vi "Main.vi"(11 "Module Admin":refnum<class "Delacor_lib_QMH_Module Admin.lvclass">) -> ()   [LabVIEW 2023, in "Registration.lvlib"]
doc: "This template is based off of the Queued Message Handler design pattern and the Queued Message Handler project template that ships with LabVIEW.\n\nThe main difference is that the queue is private to this module and communication between modules is performed via Broadcast and Request events.\n\nRequest events are wrapped in public API methods and are handled in the Event Handling Loop (EHL) of this VI. Any module can register for Broadcast events sent by this module. The EHL generates messages based on user interface actions.\n\nThe Message Handling Loop (MHL) processes messages generated by the EHL, or by other messages. The messages are string values, so new messages can be added easily to the Message Cases case structure in the MHL. Each message cluster can also provide an optional value for Message Data, which is a variant that can be converted to whatever message-specific data is required.\n_____\nBased on DQMH Project Template 6.1.0.94."
uses:
  Registration.lvlib
  <vilib>/Delacor/Delacor QMH/Libraries/Module Admin_class/Delacor_lib_QMH_Module Admin.lvclass
  Data_reg.ctl
  Module Data--cluster.ctl
  Initial Data/InitalData Type.ctl
  <vilib>/Delacor/Delacor QMH/Libraries/Message Queue_class/Delacor_lib_QMH_Message Queue.lvclass/Delacor_lib_QMH_Message Queue.ctl
  Stop Argument--cluster.ctl
  <vilib>/Delacor/Delacor QMH/Libraries/Module Admin_class/Delacor_lib_QMH_Module Admin.lvclass/Delacor_lib_QMH_Module Admin.ctl
  New_Data Argument--cluster.ctl
  Send Main VI ref Argument--cluster.ctl
  <vilib>/Utility/miscctls.llb/LVPointTypeDef.ctl
  <vilib>/Delacor/Delacor QMH/Libraries/Message Queue_class/Delacor_lib_QMH_Enqueue Message (Single).vi
  <vilib>/Delacor/Delacor QMH/Libraries/Module Admin_class/Delacor_lib_QMH_Get External Launch.vi
  <vilib>/Utility/error.llb/Error Cluster From Error Code.vi
  <vilib>/Utility/file.llb/Write Delimited Spreadsheet (string).vi
  <vilib>/ErrorRing/Error Ring.xnode
  <vilib>/Delacor/Delacor QMH/Libraries/Message Queue_class/Delacor_lib_QMH_Message Queue.lvclass
  Initial Data/Initial Data.lvlib
panel:
  in  "open_F":bool
  in  "Registr start":bool
  in  "timeout":dbl=1.0 caption="Период регистрации" format="Период регистрации %#.1f сек"
  in  "set_path":bool
  out "file_path":string caption="Файл регистрации"
  out "error out":errorcluster
  in  "Simulate MHL Error":bool
  in  "Simulate EHL Error":bool
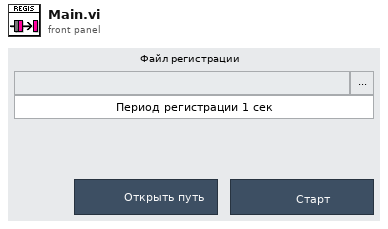
[diagram p1: front panel]
types:
  T1 = typedef "Registration.lvlib/Data_reg.ctl" = cluster{"Дата":string, "Время":string, "Рпл1, МПа":dbl, "Vпл, см3":dbl, "Рпл2, МПа":dbl, "Ргор, МПа":dbl, "Рэфф, МПа":dbl, "R, Ом":dbl, "dL, мм":dbl, "Ткд, градС":dbl, "Тпрод, мкс":dbl, "Тпоп.1, мкс":dbl, "Тпоп.2, мкс":dbl, "Рдм, МПа":dbl, "Q, мл":dbl, "Тнагр, градС":dbl, "ЦАП, градС":dbl}
  T2 = typedef "Registration.lvlib/Request Events--cluster.ctl" = cluster{"Stop Module":refnum<user-event>, "Show Panel":refnum<user-event>, "Hide Panel":refnum<user-event>, "Get Module Execution Status":refnum<user-event>, "Show Diagram":refnum<user-event>, "New_Data":refnum<user-event>, "Send Main VI ref":refnum<user-event>}
  T3 = typedef "Initial Data.lvlib/Broadcast Events--cluster.ctl" = cluster{"Module Did Init":refnum<user-event>, "Status Updated":refnum<user-event>, "Error Reported":refnum<user-event>, "Module Did Stop":refnum<user-event>, "Update Module Execution Status":refnum<user-event>, "Data":refnum<user-event>}
  T4 = typedef "Registration.lvlib/Module Data--cluster.ctl" = cluster{"reg_on":bool, "file_path":path, "Data reg":T1, "Исходные данные":T5}
  T5 = typedef "Initial Data.lvlib/InitalData Type.ctl" = cluster{"Дата":string, "Время":string, "Месторождение":string, "Пласт":string, "Скважина":string}
  T6 = enum32{"invalid lock state", "Not Locked", "Locked (No Password)", "Password-protected"}
  T7 = typedef "Registration.lvlib/Stop Argument--cluster.ctl" = cluster{"Origin":string, "Exit via Stop Module Req?":bool, "Wait for Module to stop?":bool}
  T8 = typedef "Registration.lvlib/New_Data Argument--cluster.ctl" = cluster{"Data reg":T1}
  T9 = typedef "Registration.lvlib/Send Main VI ref Argument--cluster.ctl" = cluster{"Boolean":bool}
  T10 = enum8{"Enabled", "Disabled", "Disabled and Grayed Out"}
  T11 = typedef "LVPointTypeDef.ctl" = cluster{"Horizontal":i16, "Vertical":i16}
  T12 = enum32{"Invalid", "Standard", "Closed", "Hidden", "Minimized", "Maximized"}
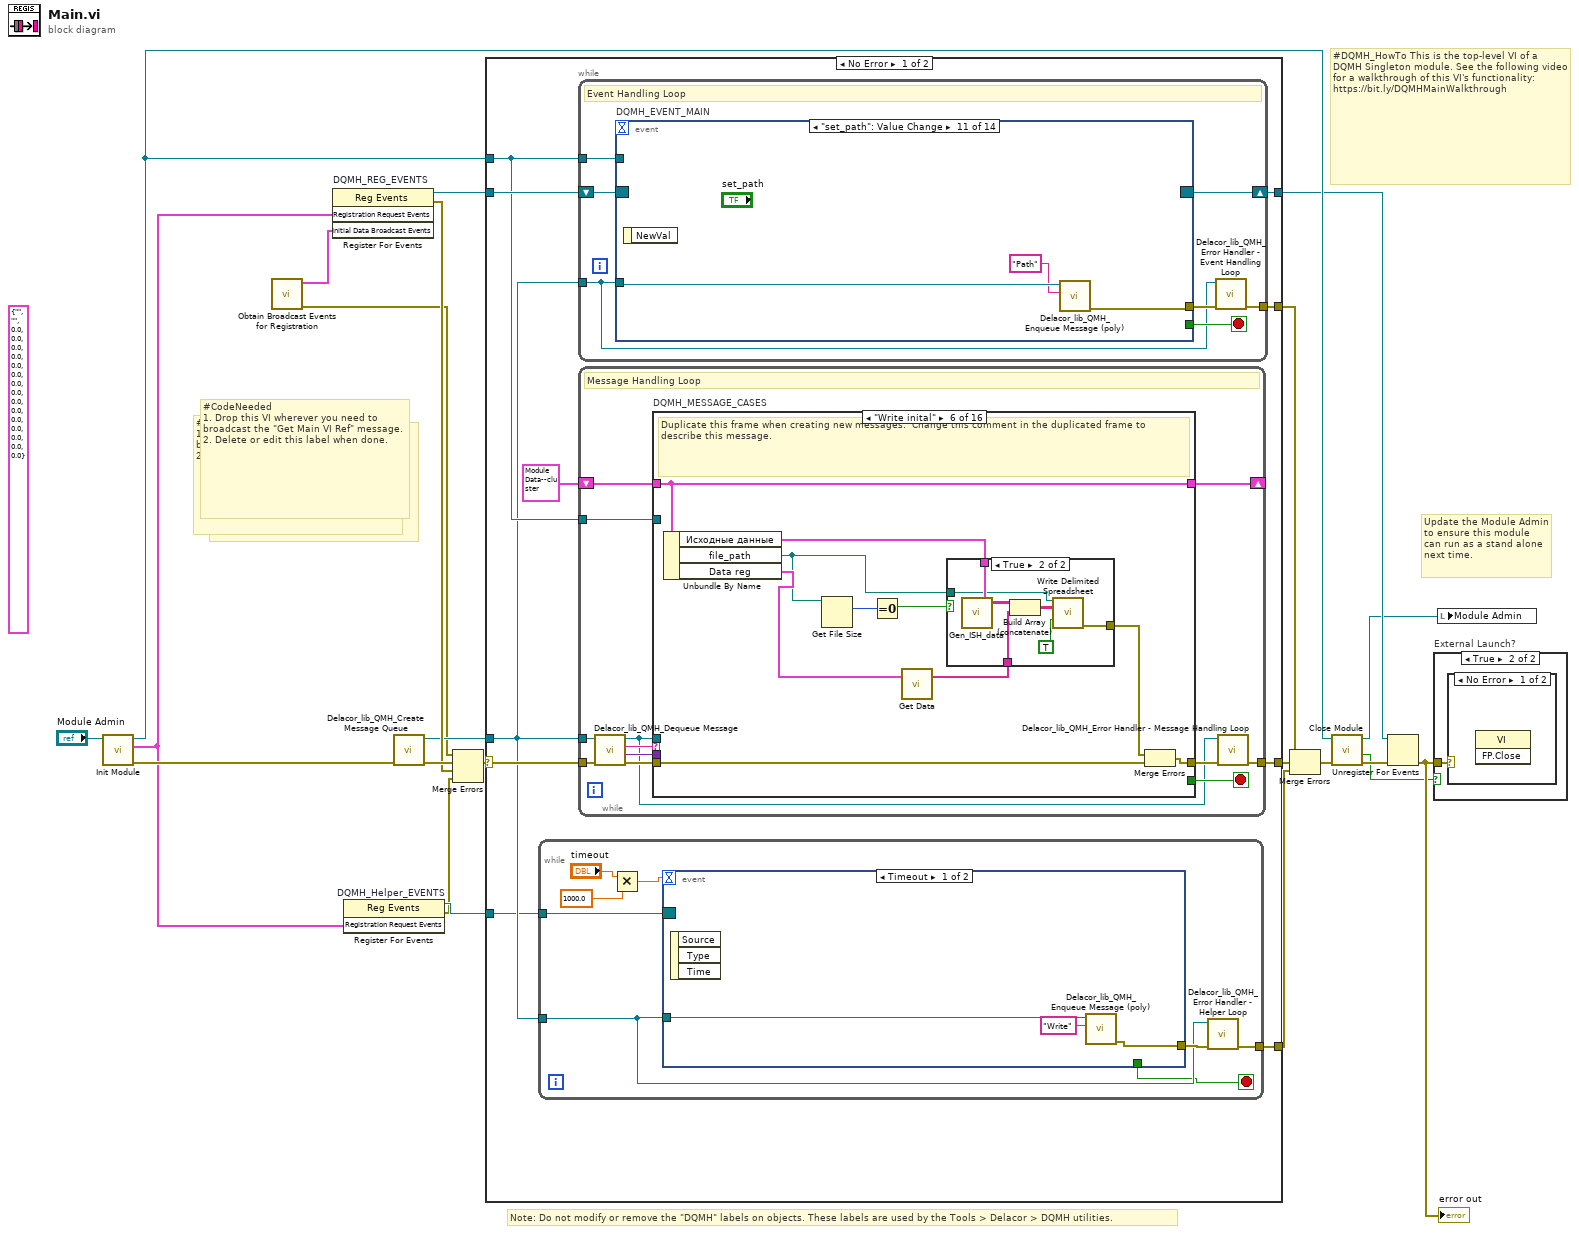
[diagram p0: block diagram]
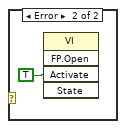
[diagram p3: hidden frame]
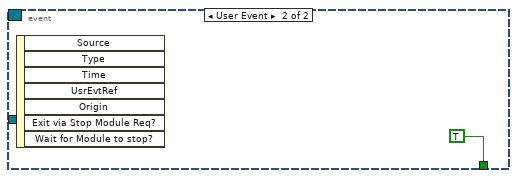
[diagram p4: hidden frame]
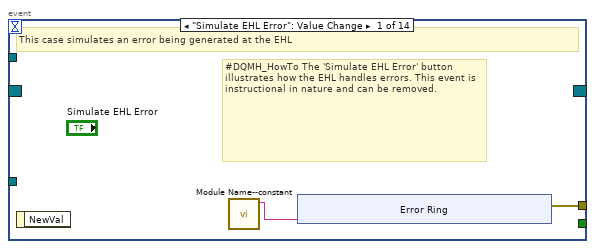
[diagram p5: hidden frame]
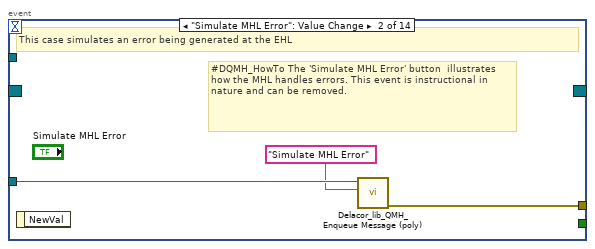
[diagram p6: hidden frame]
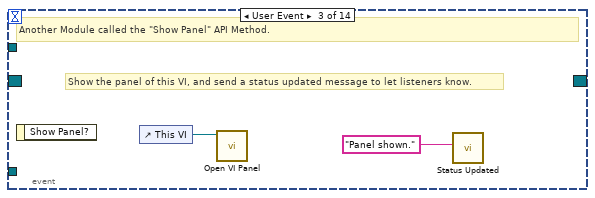
[diagram p7: hidden frame]
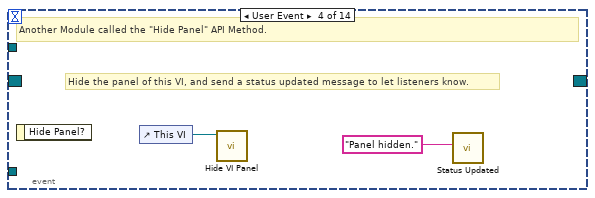
[diagram p8: hidden frame]
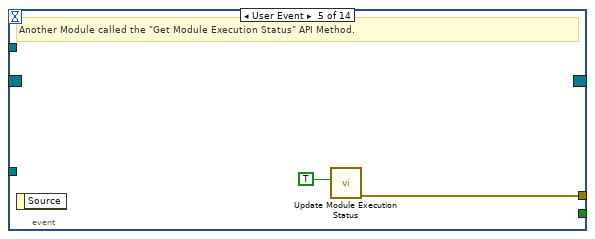
[diagram p9: hidden frame]
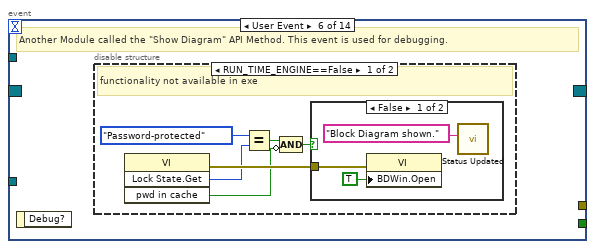
[diagram p10: hidden frame]
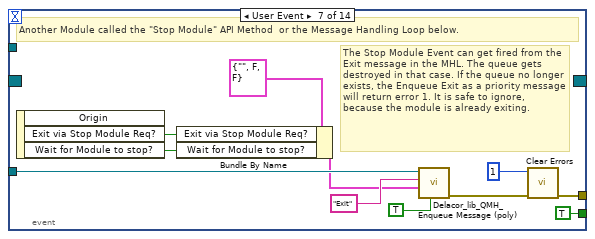
[diagram p13: hidden frame]
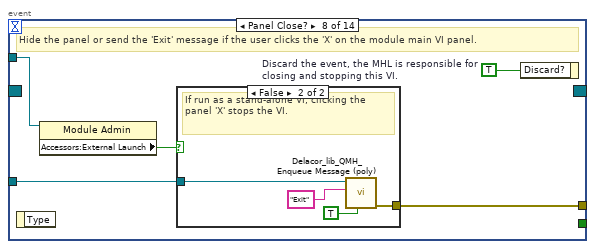
[diagram p14: hidden frame]
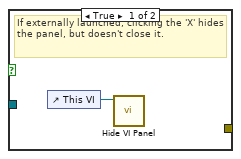
[diagram p15: hidden frame]
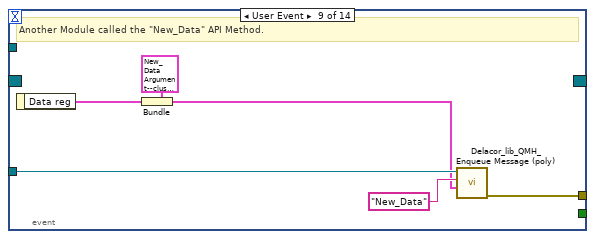
[diagram p16: hidden frame]
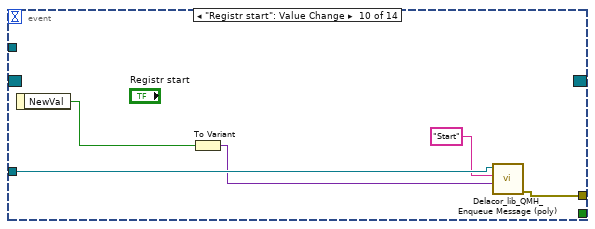
[diagram p17: hidden frame]
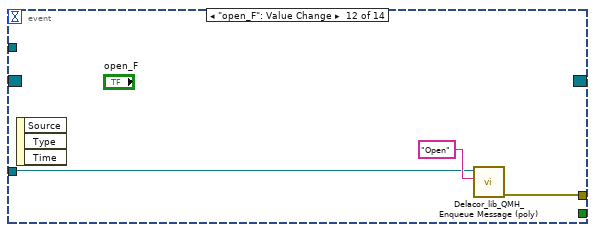
[diagram p18: hidden frame]
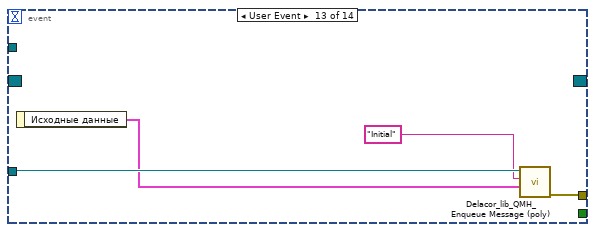
[diagram p19: hidden frame]
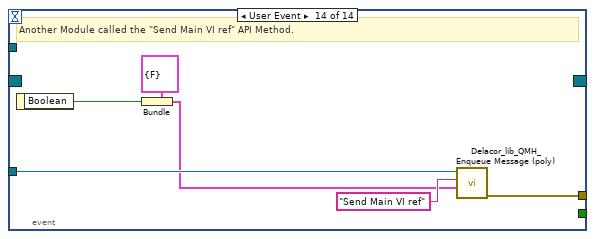
[diagram p20: hidden frame]
diagram:
  (unwired) T1 {"Дата"="", "Время"="", "Рпл1, МПа"=0.0, "Vпл, см3"=0.0, "Рпл2, МПа"=0.0, "Ргор, МПа"=0.0, "Рэфф, МПа"=0.0, "R, Ом"=0.0, "dL, мм"=0.0, "Ткд, градС"=0.0, "Тпрод, мкс"=0.0, "Тпоп.1, мкс"=0.0, "Тпоп.2, мкс"=0.0, "Рдм, МПа"=0.0, "Q, мл"=0.0, "Тнагр, градС"=0.0, "ЦАП, градС"=0.0} ("Data reg")
  # "#CodeNeeded\n1. Drop this VI wherever you need to broadcast the \"Get Main VI Reference\" message.\n2. Delete or edit this label when done."
  # "#CodeNeeded\n1. Drop this VI wherever you need to broadcast the \"Get Main VI Ref\" message.\n2. Delete or edit this label when done."
  # "#CodeNeeded\n1. Drop this VI wherever you need to broadcast the \"Get Main VI Ref\" message.\n2. Delete or edit this label when done."
  # "#DQMH_HowTo This is the top-level VI of a DQMH Singleton module. See the following video for a walkthrough of this VI's functionality: https://bit.ly/DQMHMainWalkthrough"
  # "Note: Do not modify or remove the \"DQMH\" labels on objects. These labels are used by the Tools > Delacor > DQMH utilities."
  # "Update the Module Admin to ensure this module can run as a stand alone next time."
  n1 = call "Init Module.vi"("Singleton Module Admin in"="Module Admin") -> ("error out"=w21:errorcluster, "Registration Request Events"=w1:T2, "Singleton Module Admin out"=w13:refnum<class "Delacor_lib_QMH_Module Admin.lvclass">)  [unwired: 8 in]
  n2 = call "Obtain Broadcast Events for Registration.vi"() -> ("error out"=w2:errorcluster, "Initial Data Broadcast Events"=w3:T3)  [unwired: 9 in, 1 out]
  n3 = register-events "DQMH_REG_EVENTS"(w1, w3) -> (reference out=w11:refnum<event-registration>, error out=w14:errorcluster)  [unwired: 2 in]
  n4 = register-events "DQMH_Helper_EVENTS"(w1) -> (reference out=w6:refnum<event-registration>, error out=w5:errorcluster)  [unwired: 2 in]
  n5 = call <vilib>:"Delacor_lib_QMH_Create Message Queue.vi"("error in"=w21) -> ("error out"=w16:errorcluster, "Message Queue"=w10:refnum<class "Delacor_lib_QMH_Message Queue.lvclass">)  [unwired: 9 in]
  n6 = Merge Errors(w2, w16, w14, w5) -> (w15:errorcluster)
  n7 = case shown="No Error" w15 {
    selector: w15 -> [w30 w340]
    tunnel: [w32 w339] -> w22
    tunnel: [w29 w345] -> w12
    tunnel: w11 -> [w27 w345]
    tunnel: w10 -> [w25 w338]
    tunnel: [w31 _] -> w19
    tunnel: w13 -> [w26 w341]
    tunnel: w6 -> [w24 _]
    tunnel: [w23 _] -> w4
    frame No Error {
      n8 = while {
        tunnel: w25 -> [w36]
        tunnel: w24 -> [w35]
        tunnel: [w33] -> w23
        stop <- w34 stop-if-true
        n9 = Multiply(x="timeout", y=1000.0) -> (x*y=w38:dbl)
        n10 = event shown="[0] Timeout" {
          selector: w35 -> [_ _]
          dyn-events: _ -> [_ _]
          timeout: w38 -> [_ _]
          tunnel: w36 -> [w43 _]
          tunnel: [w42 _] -> w37
          tunnel: [_ TRUE] -> w34
          event Timeout {
            n11 = event-data() -> ()  [unwired: 1 in, 3 out]
            n12 = call-poly <vilib>:"Delacor_lib_QMH_Enqueue Message (poly).vi"("Message"="Write", "Message Queue in"=w43) -> ("error out"=w42:errorcluster)  [unwired: 8 in, 1 out]
          }
          event User Event {
            n13 = event-data() -> ()  [unwired: 1 in, 7 out]
          }
        }
        n14 = call-dynamic "Delacor_lib_QMH_Error Handler - Helper Loop.vi"("error in"=w37, "Message Queue in"=w36) -> ("dup error in"=w33:errorcluster)  [unwired: 8 in, 1 out]
      }
      n15 = while {
        tunnel: w25 -> [w45]
        shift-right: [w48] -> w29
        shift-left: w27 -> [w49]
        tunnel: [w50] -> w31
        tunnel: w26 -> [w46]
        stop <- w47 stop-if-true
        # "Event Handling Loop"
        n16 = event "DQMH_EVENT_MAIN" shown="[10] \"set_path\": Value Change" {
          selector: w49 -> [_ _ _ _ _ _ _ _ _ _ _ _ _ _]
          dyn-events: [_ _ _ _ _ _ _ _ _ _ _ _ _ _] -> w48
          timeout: _ -> [_ _ _ _ _ _ _ _ _ _ _ _ _ _]
          tunnel: [_ _ _ _ _ _ TRUE ("Discard?") _ _ _ _ _ _ _] -> w47
          tunnel: w45 -> [_ w62 _ _ _ _ w85 w92 w105 w110 w112 w114 w119 w126]
          tunnel: [w53 w63 _ _ w69 _ w88 w94 w100 w109 w113 w115 w120 w121] -> w51
          tunnel: w46 -> [_ _ _ _ _ _ _ w91 _ _ _ _ _ _]
          event "Simulate EHL Error": Value Change {
            # "#DQMH_HowTo The 'Simulate EHL Error' button  illustrates how the EHL handles errors. This event is instructional in nature and can be removed."
            # "This case simulates an error being generated at the EHL"
            n17 = event-data() -> ()  [unwired: 1 in, 1 out]
            n18 = call "Module Name--constant.vi"() -> ("Module Name"=w52:string)  [unwired: 11 in]
            n19 = xnode "Error Ring"("parameter 0"=w52) -> ("error out"=w53:errorcluster)
          }
          event "Simulate MHL Error": Value Change {
            # "#DQMH_HowTo The 'Simulate MHL Error' button  illustrates how the MHL handles errors. This event is instructional in nature and can be removed."
            # "This case simulates an error being generated at the EHL"
            n20 = event-data() -> ()  [unwired: 1 in, 1 out]
            n21 = call-poly <vilib>:"Delacor_lib_QMH_Enqueue Message (poly).vi"("Message"="Simulate MHL Error", "Message Queue in"=w62) -> ("error out"=w63:errorcluster)  [unwired: 8 in, 1 out]
          }
          event User Event {
            # "Show the panel of this VI, and send a status updated message to let listeners know."
            # "Another Module called the \"Show Panel\" API Method."
            n22 = event-data() -> ()  [unwired: 1 in, 1 out]
            n23 = control-ref of="This VI"() -> (w65:refnum<vi>)
            n24 = call "Open VI Panel.vi"("VI"=w65) -> ()  [unwired: 10 in, 1 out]
            n25 = call "Status Updated.vi"("Status"="Panel shown." ("format string")) -> ()  [unwired: 10 in, 1 out]
          }
          event User Event {
            # "Hide the panel of this VI, and send a status updated message to let listeners know."
            # "Another Module called the \"Hide Panel\" API Method."
            n26 = event-data() -> ()  [unwired: 1 in, 1 out]
            n27 = control-ref of="This VI"() -> (w67:refnum<vi>)
            n28 = call "Hide VI Panel.vi"("VI"=w67) -> ()  [unwired: 10 in, 1 out]
            n29 = call "Status Updated.vi"("Status"="Panel hidden." ("format string")) -> ()  [unwired: 10 in, 1 out]
          }
          event User Event {
            # "Another Module called the \"Get Module Execution Status\" API Method."
            n30 = event-data() -> ()  [unwired: 1 in, 1 out]
            n31 = call "Update Module Execution Status.vi"("Running?"=TRUE) -> ("error out"=w69:errorcluster)  [unwired: 10 in]
          }
          event User Event {
            # "Another Module called the \"Show Diagram\" API Method. This event is used for debugging."
            n32 = event-data() -> ()  [unwired: 1 in, 1 out]
            n33 = disable-structure shown="RUN_TIME_ENGINE==False" {
              frame condition #0 (active) {
                # "functionality not available in exe"
                n34 = invoke class="VI" method="Lock State.Get"() -> (error out=w75:errorcluster, "Get Lock State"=w74:T6, "pwd in cache"=w71:bool)  [unwired: 4 in, 1 out]
                n35 = Equal?(x=T6."Password-protected", y=w74) -> (x = y?=w72:bool)
                n36 = Compound Arithmetic op=AND(w72, invert w71) -> (w70:bool)
                n37 = case shown="False" w70 {
                  tunnel: w75 -> [w78 _]
                  frame False {
                    n38 = property class="VI"(error in=w78, "BDWin.Open"=TRUE ("Block Diagram Window:Open")) -> ()  [unwired: 1 in, 2 out]
                    n39 = call "Status Updated.vi"("Status"="Block Diagram shown." ("format string")) -> ()  [unwired: 10 in, 1 out]
                  }
                  frame True {
                    # "Password-protected VI, and the password is not in the cache. Do not show the diagram."
                  }
                }
              }
              frame condition #1 {
              }
            }
          }
          event User Event {
            # "The Stop Module Event can get fired from the Exit message in the MHL. The queue gets destroyed in that case. If the queue no longer exists, the Enqueue Exit as a priority message will return error 1. It is safe to ignore, because the module is already exiting."
            # "Another Module called the \"Stop Module\" API Method  or the Message Handling Loop below."
            n40 = event-data() -> ("Exit via Stop Module Req?"=w81:bool, "Wait for Module to stop?"=w80:bool)  [unwired: 1 in, 1 out]
            n41 = Bundle By Name(cluster=T7 {"Origin"="", "Exit via Stop Module Req?"=FALSE, "Wait for Module to stop?"=FALSE} ("Stop Argument"), "Exit via Stop Module Req?"=w81, "Wait for Module to stop?"=w80) -> (w79:T7)
            n42 = call-poly <vilib>:"Delacor_lib_QMH_Enqueue Message (poly).vi"("Priority Message? (F)"=TRUE, "Message Data"=w79, "Message"="Exit", "Message Queue in"=w85) -> ("error out"=w89:errorcluster)  [unwired: 6 in, 1 out]
            n43 = call <vilib>:"Clear Errors.vi"("error in (no error)"=w89, "specific error code to clear (0: all)"=1) -> ("error out"=w88:errorcluster)  [unwired: 4 in, 1 out]
          }
          event Panel Close? {
            w93 = TRUE  # Discard the event, the MHL is responsible for closing and stopping this VI.
            # "Hide the panel or send the 'Exit' message if the user clicks the 'X' on the module main VI panel."
            n44 = event-data() -> ()  [unwired: 1 in, 1 out]
            n45 = property class="Module Admin"(reference=w91) -> ("Accessors:External Launch"=w90:bool)  [unwired: 1 in, 2 out]
            n46 = case shown="False" w90 {
              tunnel: w92 -> [_ w98]
              tunnel: [_ w99] -> w94
              frame True {
                # "If externally launched, clicking the 'X' hides the panel, but doesn't close it."
                n47 = control-ref of="This VI"() -> (w95:refnum<vi>)
                n48 = call "Hide VI Panel.vi"("VI"=w95) -> ()  [unwired: 10 in, 1 out]
              }
              frame False {
                # "If run as a stand-alone VI, clicking the panel 'X' stops the VI."
                n49 = call-poly <vilib>:"Delacor_lib_QMH_Enqueue Message (poly).vi"("Priority Message? (F)"=TRUE, "Message"="Exit", "Message Queue in"=w98) -> ("error out"=w99:errorcluster)  [unwired: 7 in, 1 out]
              }
            }
            n50 = event-data("Discard?"=w93) -> ()  [unwired: 1 in, 1 out]
          }
          event User Event {
            # "Another Module called the \"New_Data\" API Method."
            n51 = event-data() -> ("Data reg"=w101:T1)  [unwired: 1 in]
            n52 = Bundle(cluster=T8 {"Data reg"={"Дата"="", "Время"="", "Рпл1, МПа"=0.0, "Vпл, см3"=0.0, "Рпл2, МПа"=0.0, "Ргор, МПа"=0.0, "Рэфф, МПа"=0.0, "R, Ом"=0.0, "dL, мм"=0.0, "Ткд, градС"=0.0, "Тпрод, мкс"=0.0, "Тпоп.1, мкс"=0.0, "Тпоп.2, мкс"=0.0, "Рдм, МПа"=0.0, "Q, мл"=0.0, "Тнагр, градС"=0.0, "ЦАП, градС"=0.0}} ("New_Data Argument"), "Data reg"=w101) -> (w102:T8)
            n53 = call-poly <vilib>:"Delacor_lib_QMH_Enqueue Message (poly).vi"("Message Data"=w102, "Message"="New_Data", "Message Queue in"=w105) -> ("error out"=w100:errorcluster)  [unwired: 7 in, 1 out]
          }
          event "Registr start": Value Change {
            n54 = event-data() -> ("NewVal"=w107:bool)  [unwired: 1 in]
            n55 = To Variant(anything=w107) -> (Variant=w106:variant)
            n56 = call-poly <vilib>:"Delacor_lib_QMH_Enqueue Message (poly).vi"("Message Data"=w106, "Message"="Start", "Message Queue in"=w110) -> ("error out"=w109:errorcluster)  [unwired: 7 in, 1 out]
          }
          event "set_path": Value Change {
            n57 = event-data() -> ()  [unwired: 1 in, 1 out]
            n58 = call-poly <vilib>:"Delacor_lib_QMH_Enqueue Message (poly).vi"("Message"="Path", "Message Queue in"=w112) -> ("error out"=w113:errorcluster)  [unwired: 8 in, 1 out]
          }
          event "open_F": Value Change {
            n59 = event-data() -> ()  [unwired: 1 in, 3 out]
            n60 = call-poly <vilib>:"Delacor_lib_QMH_Enqueue Message (poly).vi"("Message"="Open", "Message Queue in"=w114) -> ("error out"=w115:errorcluster)  [unwired: 8 in, 1 out]
          }
          event User Event {
            n61 = event-data() -> ("Исходные данные"=w118:T5)  [unwired: 1 in]
            n62 = call-poly <vilib>:"Delacor_lib_QMH_Enqueue Message (poly).vi"("Message Data"=w118, "Message"="Initial", "Message Queue in"=w119) -> ("error out"=w120:errorcluster)  [unwired: 7 in, 1 out]
          }
          event User Event {
            # "Another Module called the \"Send Main VI ref\" API Method."
            n63 = event-data() -> ("Boolean"=w122:bool)  [unwired: 1 in]
            n64 = Bundle(cluster=T9 {"Boolean"=FALSE} ("Send Main VI ref Argument"), "Boolean"=w122) -> (w123:T9)
            n65 = call-poly <vilib>:"Delacor_lib_QMH_Enqueue Message (poly).vi"("Message Data"=w123, "Message"="Send Main VI ref", "Message Queue in"=w126) -> ("error out"=w121:errorcluster)  [unwired: 7 in, 1 out]
          }
        }
        n66 = call-dynamic "Delacor_lib_QMH_Error Handler - Event Handling Loop.vi"("error in"=w51, "Message Queue in"=w45) -> ("dup error in"=w50:errorcluster)  [unwired: 8 in, 1 out]
      }
      n67 = while {
        tunnel: w25 -> [w129]
        shift-right: [w133] -> _
        shift-left: T4 {"reg_on"=FALSE, "file_path"=path "", "Data reg"={"Дата"="", "Время"="", "Рпл1, МПа"=0.0, "Vпл, см3"=0.0, "Рпл2, МПа"=0.0, "Ргор, МПа"=0.0, "Рэфф, МПа"=0.0, "R, Ом"=0.0, "dL, мм"=0.0, "Ткд, градС"=0.0, "Тпрод, мкс"=0.0, "Тпоп.1, мкс"=0.0, "Тпоп.2, мкс"=0.0, "Рдм, МПа"=0.0, "Q, мл"=0.0, "Тнагр, градС"=0.0, "ЦАП, градС"=0.0}, "Исходные данные"={"Дата"="", "Время"="", "Месторождение"="", "Пласт"="", "Скважина"=""}} ("Data Cluster") -> [w134]
        tunnel: w30 -> [w137]
        tunnel: [w135] -> w32
        tunnel: w26 -> [w127]
        stop <- w132 stop-if-true
        # "Message Handling Loop"
        n68 = call-dynamic "Delacor_lib_QMH_Dequeue Message.vi"("error in"=w137, "Message Queue in"=w129) -> ("error out"=w136:errorcluster, "Message Data"=w130:variant, "Message"=w131:string, "Message Queue out"=w128:refnum<class "Delacor_lib_QMH_Message Queue.lvclass">)  [unwired: 6 in]
        n69 = case "DQMH_MESSAGE_CASES" shown="\"Write inital\"" w131 {
          selector: w131 -> [_ _ _ _ _ _ _ _ _ _ _ _ _ _ _ w325]
          tunnel: w128 -> [_ _ _ _ _ _ _ _ _ _ w267 _ _ w295 w317 _]
          tunnel: w136 -> [w155 w159 w173 w181 w184 w194 w209 w220 w230 w258 w276 w280 w285 w302 w323 w327]
          tunnel: [w153 w159 w171 w174 w183 w193 w208 w219 w229 w257 w278 w280 w284 w298 w320 w328] -> w138
          tunnel: w134 -> [w146 w158 w172 w180 w182 w192 w207 w215 w228 w256 w272 w279 w282 w297 w316 w326]
          tunnel: [w146 w158 w167 w180 w182 w192 w205 w215 w228 w255 w277 w279 w282 w297 w316 w326] -> w133
          tunnel: [_ _ _ _ _ _ _ _ _ _ _ _ _ _ w315 _] -> w132
          tunnel: w130 -> [_ _ w170 w179 _ _ w206 _ _ _ w274 _ _ w296 w314 _]
          tunnel: w127 -> [w147 _ _ _ _ _ _ _ _ _ _ _ _ w294 w309 _]
          frame "Initialize" {
            # "Initialize - Any operation that needs to be done before the module can receive messages. Synchronize Caller Events.vi will inform Start Module.vi that the module has launched and is ready to receive messages. Module Did Init.vi will broadcast that the module initialized."
            n70 = call "Synchronize Caller Events.vi"("error in (no error)"=w155, "Singleton Module Admin in"=w147) -> ("error out"=w154:errorcluster, "Singleton Module Admin out"=w143:refnum<class "Delacor_lib_QMH_Module Admin.lvclass">)  [unwired: 8 in]
            n71 = disable-structure shown="Disabled" {
              frame Disabled {
                n72 = control-ref of="This VI"() -> (w157:refnum<vi>)
                n73 = call "ShowBar.vi"("This VI"=w157) -> ()
              }
              frame Enabled {
              }
            }
            n74 = property class="Module Admin"(reference=w143) -> ("Accessors:External Launch"=w151:bool)  [unwired: 1 in, 2 out]
            n75 = Select(t=T12."Hidden" ("State"), s=w151, f=T12."Standard" ("State")) -> (s? t:f=w148:T12)
            n76 = local write "file_path"("" ("file_path")) -> ()
            n77 = property on="Registr start" class="Bool (strict)"("DisabledEnum"=T10."Disabled and Grayed Out" ("Disabled")) -> ()  [unwired: 2 in, 2 out]
            n78 = property class="VI"("Front Panel.Title"="Управление регистрацией" ("Front Panel Window:Title")) -> (reference out=w152:refnum<vi>, error out=w156:errorcluster)  [unwired: 2 in]
            n79 = call "Module Name--constant.vi"() -> ("Module Name"=w144:string)  [unwired: 11 in]
            n80 = invoke class="VI" method="FP.Open"(reference=w152, error in=w156, "State"=w148) -> ()  [unwired: 2 in, 5 out]
            n81 = call "Module Did Init.vi"("error in (no error)"=w154, "Initialized?"=TRUE, "Origin"=w144) -> ("error out"=w153:errorcluster)  [unwired: 8 in]
            n82 = property on="Pane" class="Pane"("Origin"=T11 {"Horizontal"=0, "Vertical"=0}) -> ()  [unwired: 2 in, 2 out]
          }
          frame "---Module Specific---" {
            # "Separator -- The following cases handle messages specific to this Module."
          }
          frame "New_Data" {
            n83 = Variant To Data(error in=w173, type=T8 {"Data reg"={"Дата"="", "Время"="", "Рпл1, МПа"=0.0, "Vпл, см3"=0.0, "Рпл2, МПа"=0.0, "Ргор, МПа"=0.0, "Рэфф, МПа"=0.0, "R, Ом"=0.0, "dL, мм"=0.0, "Ткд, градС"=0.0, "Тпрод, мкс"=0.0, "Тпоп.1, мкс"=0.0, "Тпоп.2, мкс"=0.0, "Рдм, МПа"=0.0, "Q, мл"=0.0, "Тнагр, градС"=0.0, "ЦАП, градС"=0.0}} ("New_Data Argument"), Variant=w170) -> (data=w168:T8, error out=w171:errorcluster)
            n84 = Unbundle By Name(w168) -> ("Data reg"=w166:T1)
            n85 = Get Date/Time In Seconds() -> (seconds since 1Jan1904=w164:timestamp)
            n86 = Get Date/Time String(date format (0)=enum16{"short", "long", "abbreviated"}."short", seconds (now)=w164, want seconds? (F)=TRUE) -> (date string=w161:string, time string=w160:string)
            n87 = Bundle By Name(cluster=w166, "Дата"=w161, "Время"=w160) -> (w165:T1)
            n88 = Bundle By Name(cluster=w172, "Data reg"=w165) -> (w167:T4)
          }
          frame "Send Main VI ref" {
            # "#CodeNeeded\n1. Configure this Message Case for handling the \"Send Main VI ref\" message.\n2. Delete or edit this label when done."
            n89 = Variant To Data(error in=w181, type=T9 {"Boolean"=FALSE} ("Send Main VI ref Argument"), Variant=w179) -> (data=w177:T9, error out=w175:errorcluster)
            n90 = Unbundle By Name(w177) -> ()  [unwired: 1 out]
            n91 = control-ref of="This VI"() -> (w176:refnum<vi>)
            n92 = call "Get Main VI Reference.vi"("error in"=w175, "VI Refnum"=w176) -> ("error out"=w174:errorcluster)  [unwired: 9 in]
          }
          frame "---Copy This Frame---" {
            # "Duplicate this frame when creating new messages.  Change this comment in the duplicated frame to describe this message."
            n93 = Merge Errors(w184) -> (w183:errorcluster)
          }
          frame "Write inital" {
            # "Duplicate this frame when creating new messages.  Change this comment in the duplicated frame to describe this message."
            n94 = Unbundle By Name(w192) -> ("Исходные данные"=w188:T5, "file_path"=w185:path, "Data reg"=w187:T1)
            n95 = Get File Size(file=w185) -> (size (in bytes)=w191:i64)  [unwired: 1 in, 2 out]
            n96 = Equal To 0?(x=w191) -> (x = 0?=w189:bool)
            n97 = call "Get Data.vi"("Data reg"=w187) -> ("Array of Headers"=w186:string[])  [unwired: 1 in, 1 out]
            n98 = case shown="True" w189 {
              tunnel: [_ w201] -> w190
              tunnel: w188 -> [_ w199]
              tunnel: w186 -> [_ w196]
              tunnel: w185 -> [_ w197]
              frame False {
              }
              frame True {
                n99 = call "Gen_ISH_data.vi"("Исходные данные"=w199) -> ("Исходные tbl"=w200:string[][])  [unwired: 4 in]
                n100 = Build Array (concatenate)(w200, w196) -> (w195:string[][])
                n101 = call-poly <vilib>:"Write Delimited Spreadsheet.vi"("file path (dialog if empty)"=w197, "2D data"=w195, "append to file? (new file:F)"=TRUE) -> ("error out"=w201:errorcluster)  [unwired: 11 in, 1 out]
              }
            }
            n102 = Merge Errors(w190, w194) -> (w193:errorcluster)
          }
          frame "Initial" {
            # "Duplicate this frame when creating new messages.  Change this comment in the duplicated frame to describe this message."
            n103 = Variant To Data(type=T5 {"Дата"="", "Время"="", "Месторождение"="", "Пласт"="", "Скважина"=""} ("Исходные данные"), Variant=w206) -> (data=w204:T5, error out=w203:errorcluster)  [unwired: 1 in]
            n104 = Bundle By Name(cluster=w207, "Исходные данные"=w204) -> (w205:T4)
            n105 = Merge Errors(w203, w209) -> (w208:errorcluster)
          }
          frame "Open" {
            w213 = "\""
            # "Duplicate this frame when creating new messages.  Change this comment in the duplicated frame to describe this message."
            n106 = Unbundle By Name(w215) -> ("file_path"=w211:path)
            n107 = Strip Path(path=w211) -> (stripped path=w210:path)  [unwired: 1 out]
            n108 = Path To String(path=w210) -> (string=w214:string)
            n109 = Concatenate Strings(w213, w214, w213) -> (w212:string)
            n110 = Concatenate Strings("explorer.exe " ("command line"), w212) -> (w216:string)
            n111 = call <vilib>:"System Exec.vi"("command line"=w216) -> ("error out"=w218:errorcluster)  [unwired: 7 in, 3 out]
            n112 = Merge Errors(w218, w220) -> (w219:errorcluster)
          }
          frame "Write" {
            # "Duplicate this frame when creating new messages.  Change this comment in the duplicated frame to describe this message."
            n113 = Unbundle By Name(w228) -> ("reg_on"=w226:bool, "file_path"=w225:path, "Data reg"=w227:T1)
            n114 = call "Get Data.vi"("Data reg"=w227) -> ("Array of Data"=w224:string[], "Array of Headers"=w222:string[])  [unwired: 1 in]
            n115 = for {
              tunnel: w222 -> [w237] mode=indexing
              tunnel: [w234] -> w221 mode=indexing
              n116 = Search and Replace String(replace all?=TRUE ("replace all? (F)"), input string=w237, search string="\n", replace string=" " ("replace string (\"\")"), error in=errorcluster {"status"=FALSE, "code"=0, "source"=""} ("error in (no error)")) -> (result string=w234:string, error out=w235:errorcluster)  [unwired: 3 in, 2 out]
              n117 = Unbundle(w235) -> ()  [unwired: 3 out]
            }
            n118 = case shown="True" w226 {
              tunnel: w225 -> [w238 w242]
              tunnel: w221 -> [_ w249]
              tunnel: w224 -> [_ w246]
              tunnel: [w238 w240] -> _
              tunnel: [_ w239] -> w223
              frame False {
              }
              frame True {
                n119 = Get File Size(file=w242) -> (size (in bytes)=w250:i64, 0:w243:errorcluster)  [unwired: 1 in, 1 out]
                n120 = Build Array(w246) -> (w245:string[][])
                n121 = Build Array(w249, w246) -> (w247:string[][])
                n122 = Equal To 0?(x=w250) -> (x = 0?=w248:bool)
                n123 = Select(t=w247, s=w248, f=w245) -> (s? t:f=w244:string[][])
                n124 = call-poly <vilib>:"Write Delimited Spreadsheet.vi"("file path (dialog if empty)"=w242, "2D data"=w244, "append to file? (new file:F)"=TRUE, "error in (no error)"=w243) -> ("new file path (Not A Path if cancelled)"=w240:path, "error out"=w239:errorcluster)  [unwired: 10 in]
              }
            }
            n125 = Merge Errors(w223, w230) -> (w229:errorcluster)
          }
          frame "Path" {
            # "Duplicate this frame when creating new messages.  Change this comment in the duplicated frame to describe this message."
            n126 = call "Path.vi"() -> ("error out 2"=w252:errorcluster, "cancelled"=w254:bool, "selected path"=w253:path)  [unwired: 9 in]
            n127 = case shown="False" w254 {
              tunnel: w256 -> [w263 w265]
              tunnel: [w262 w265] -> w255
              tunnel: w253 -> [w260 _]
              tunnel: [T10."Enabled" ("Disabled") T10."Disabled and Grayed Out" ("Disabled")] -> w251
              frame False {
                n128 = Path To String(path=w260) -> (string=→"file_path":string)
                n129 = Bundle By Name(cluster=w263, "file_path"=w260) -> (w262:T4)
              }
              frame True {
              }
            }
            n130 = property on="Registr start" class="Bool (strict)"("DisabledEnum"=w251) -> ()  [unwired: 2 in, 2 out]
            n131 = Merge Errors(w252, w258) -> (w257:errorcluster)
          }
          frame "Start" {
            # "Duplicate this frame when creating new messages.  Change this comment in the duplicated frame to describe this message."
            n132 = Unbundle By Name(w272) -> ("file_path"=w271:path)
            n133 = Variant To Data(error in=w276, type=TRUE, Variant=w274) -> (data=w273:bool, error out=w270:errorcluster)
            n134 = call-poly <vilib>:"Delacor_lib_QMH_Enqueue Message (poly).vi"("Message"="Write inital", "Message Queue in"=w267) -> ("error out"=w268:errorcluster)  [unwired: 8 in, 1 out]
            n135 = Bundle By Name(cluster=w272, "reg_on"=w273) -> (w277:T4)
            n136 = call "Data from Registration.vi"("Path"=w271, "Registration_on"=w273) -> ("error out"=w269:errorcluster)  [unwired: 9 in]
            n137 = Merge Errors(w268, w269, w270) -> (w278:errorcluster)
          }
          frame "---Exit and Error Handling---" {
            # "Separator - The following cases handle errors and exit messages."
          }
          frame "Simulate MHL Error" {
            # "#DQMH_HowTo The 'Simulate MHL Error' button  illustrates how the MHL handles errors. This event is instructional in nature and can be removed."
            # "Simulate an error occurring at the MHL"
            n138 = call "Module Name--constant.vi"() -> ("Module Name"=w281:string)  [unwired: 11 in]
            n139 = xnode "Error Ring"("parameter 0"=w281) -> ("error out"=w283:errorcluster)
            n140 = Merge Errors(w285, w283) -> (w284:errorcluster)
          }
          frame "Error" {
            # "#CodeRecommended - If you ever change the name of this \"Error\" message, you'll need to update the name in the Check Loop Error.vi as well."
            # "#CodeRecommended - If the module is running in standalone mode (External Launch = FALSE), this code will pop up an error dialog and call the 'Exit' message if an error occurs. Add more fine-grained error handling here."
            # "Error - Check the error message data and respond accordingly. This message is sent by the \"Error Handler\" VIs at the end of each loop in this application."
            n141 = property class="Module Admin"(reference=w294) -> ("Accessors:External Launch"=w293:bool)  [unwired: 1 in, 2 out]
            n142 = Variant To Data(error in=w302, type=errorcluster {"status"=FALSE, "code"=0, "source"=""} ("error constant"), Variant=w296) -> (data=w303:errorcluster, error out=w300:errorcluster)
            n143 = call "Error Reported.vi"("Error"=w303) -> ()  [unwired: 10 in, 1 out]
            n144 = case shown="False" w293 {
              tunnel: [w308 _] -> w299
              tunnel: w295 -> [w306 _]
              tunnel: w303 -> [w307 _]
              frame False {
                # "If the module is running standalone, then pop up an error dialog and call the \"Exit\" message."
                n145 = call <vilib>:"Simple Error Handler.vi"("error in (no error)"=w307) -> ()  [unwired: 4 in, 5 out]
                n146 = call-poly <vilib>:"Delacor_lib_QMH_Enqueue Message (poly).vi"("Priority Message? (F)"=TRUE, "Message"="Exit", "Message Queue in"=w306) -> ("error out"=w308:errorcluster)  [unwired: 7 in, 1 out]
              }
              frame True {
                # "If the module was launched externally, calling the Error Reported broadcast VI is the only action performed by the \"Error\" message. The module's caller can then process the error appropriately."
              }
            }
            n147 = Merge Errors(w300, w299) -> (w298:errorcluster)
            n148 = local write "error out"(w298) -> ()
          }
          frame "Exit" {
            w313 = 91  # 91: not all Exit messages will have an argument
            w315 = TRUE  # Stop the VI
            # "Release the message queue reference"
            # "#CodeNeeded - Add any required cleanup code here"
            # "Exit - Exit the application."
            n149 = Variant To Data(error in=w323, type=T7 {"Origin"="", "Exit via Stop Module Req?"=FALSE, "Wait for Module to stop?"=FALSE} ("Stop Argument"), Variant=w314) -> (data=w311:T7, error out=w319:errorcluster)
            n150 = call <vilib>:"Clear Errors.vi"("error in (no error)"=w319, "specific error code to clear (0: all)"=w313) -> ("error out"=w322:errorcluster)  [unwired: 4 in, 1 out]
            n151 = control-ref of="This VI"() -> (w310:refnum<vi>)
            n152 = call-dynamic "Delacor_lib_QMH_Release Message Queue.vi"("error in"=w322, "Message Queue"=w317) -> ("error out"=w321:errorcluster)  [unwired: 9 in]
            n153 = call "Handle Exit.vi"("Stop Argument"=w311, "Admin in"=w309, "VI reference"=w310) -> ("error out"=w318:errorcluster)  [unwired: 7 in, 1 out]
            n154 = Merge Errors(w321, w318) -> (w320:errorcluster)
          }
          frame Default {
            # "'Default' case only runs if there is a message that isn't defined in any of the other cases.  Output a programming error."
            n155 = call "Module Name--constant.vi"() -> ("Module Name"=w324:string)  [unwired: 11 in]
            n156 = xnode "Error Ring"("parameter 0"=w325, "parameter 1"=w324) -> ("error out"=w329:errorcluster)
            n157 = Merge Errors(w327, w329) -> (w328:errorcluster)
          }
        }
        n158 = call-dynamic "Delacor_lib_QMH_Error Handler - Message Handling Loop.vi"("error in"=w138, "Message Queue in"=w128) -> ("dup error in"=w135:errorcluster)  [unwired: 8 in, 1 out]
      }
    }
    frame Error {
      # "Synchronize Caller Events.vi will inform Start Module.vi that the module has launched and will let the code calling Start Module.vi register for broadcasts and would permit the caller receive the broadcast that an error occurred at launch time."
      n159 = call-dynamic "Delacor_lib_QMH_Release Message Queue.vi"("error in"=w340, "Message Queue"=w338) -> ("error out"=w339:errorcluster)  [unwired: 9 in]
      n160 = call "Synchronize Caller Events.vi"("Singleton Module Admin in"=w341) -> ("error out"=w346:errorcluster)  [unwired: 9 in, 1 out]
      n161 = call "Module Name--constant.vi"() -> ("Module Name"=w344:string)  [unwired: 11 in]
      n162 = Format Into String(format string="An error occurred during initialization. %s is no longer running.", w344) -> (resulting string=w342:string)  [unwired: 2 in, 1 out]
      n163 = Merge Errors(w339, w346) -> (w347:errorcluster)
      n164 = call "Error Reported.vi"("Additional Information"=w342, "Error"=w347) -> ()  [unwired: 9 in, 1 out]
    }
  }
  n165 = Merge Errors(w19, w22, w4) -> (w18:errorcluster)
  n166 = call "Close Module.vi"("error in (no error)"=w18, "Module Admin in"=w13) -> ("error out"=w20:errorcluster, "External Launch"=w7:bool, "Module Admin out"=w8:refnum<class "Delacor_lib_QMH_Module Admin.lvclass">)  [unwired: 7 in]
  n167 = Unregister For Events(event registration refnum=w12, error in=w20) -> (error out=w17:errorcluster)
  "error out" <- w17
  n168 = case "External Launch?" shown="True" w7 {
    tunnel: w17 -> [_ w348]
    frame False {
    }
    frame True {
      n169 = case shown="No Error" w348 {
        frame No Error {
          n170 = invoke class="VI" method="FP.Close"() -> ()  [unwired: 3 in, 3 out]
        }
        frame Error {
          n171 = invoke class="VI" method="FP.Open"("Activate"=TRUE ("Activate?")) -> ()  [unwired: 4 in, 5 out]
        }
      }
    }
  }
  n172 = local write "Module Admin"(w8) -> ()
